vi "Maxi Gauge-RW Sensor Control.vi"(0 "VISA-Ressource in":refnum<visa-resource-name>, 1 "No Control ID´s":string[](array[string])=["no Sensor", "APR/ACR", "TPR"], 2 "Sensor Nr. :":u8(ring) items=["sensor 1", "sensor 2", "sensor 3", "sensor 4", "sensor 5", "sensor 6"], 3 "Control Source ON:":u8(ring) items=["sensor 1", "sensor 2", "sensor 3", "sensor 4", "sensor 5", "sensor 6", "Extern", "Manual", "Hotstart"], 4 "Control Source OFF:":u8(ring) items=["sensor 1", "sensor 2", "sensor 3", "sensor 4", "sensor 5", "sensor 6", "Extern", "Manual", "Hotstart"], 5 "Fehler (Eingang, kein Fehler)":errorcluster, 6 "Node address":i8=-1 min=-1 max=31 step=1, 7 "ON Threshold Set:":dbl=1e-13 min=1e-13 max=41000.0 format="%.2e", 8 "W/R":bool, 9 "OFF Threshold Set:":dbl=1e-13 min=1e-13 max=41000.0 format="%.2e") -> (14 "VISA-Ressource out":refnum<visa-resource-name>, 15 "Control Sensor ON Get:":u8(ring) items=["sensor 1", "sensor 2", "sensor 3", "sensor 4", "sensor 5", "sensor 6", "Extern", "Manual", "Hotstart"], 16 "Control Sensor OFF Get:":u8(ring) items=["sensor 1", "sensor 2", "sensor 3", "sensor 4", "sensor 5", "sensor 6", "Extern", "Manual", "Hotstart"], 17 "ON Threshold Get:":dbl=1e-13 min=1e-13 max=41000.0 format="%.2e", 18 "OFF Threshold Get:":dbl=1e-13 min=1e-13 max=41000.0 format="%.2e", 19 "Fehler (Ausgang)":errorcluster)   [LabVIEW 2012, in "Maxi Gauge.lvlib"]
uses:
  Maxi Gauge.lvlib
panel:
  # "mbar"
  # "mbar"
  # "mbar"
  # "mbar"
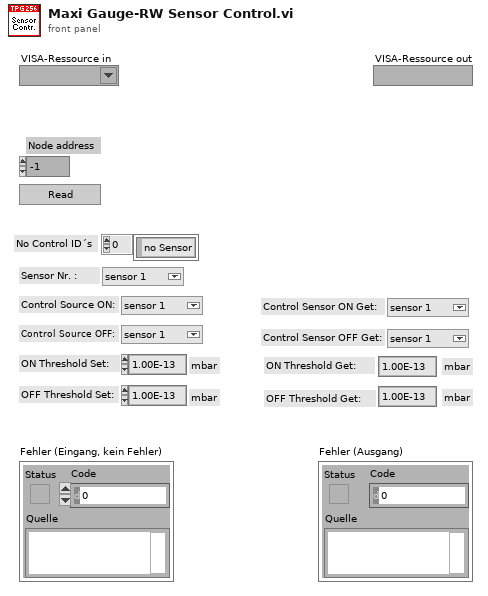
[diagram p1: front panel]
types:
  T1 = cluster{"Sensor 1":string, "Sensor 2":string, "Sensor 3":string, "Sensor 4":string, "Sensor 5":string, "Sensor 6":string}
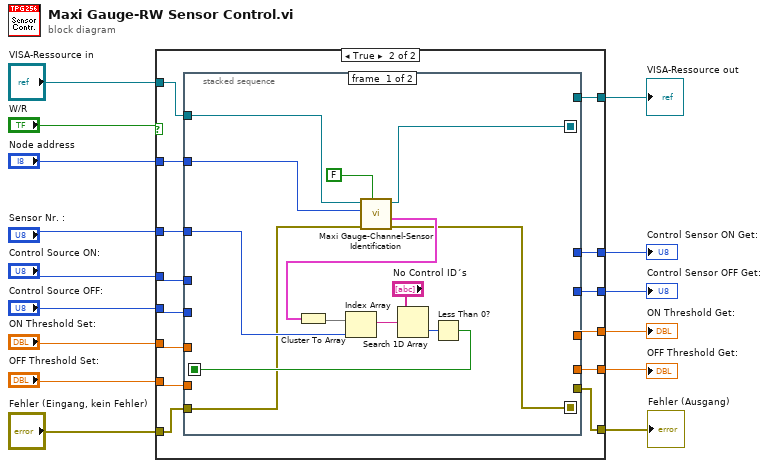
[diagram p0: block diagram]
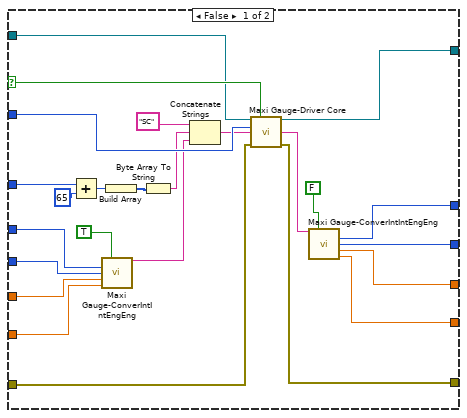
[diagram p2: hidden frame]
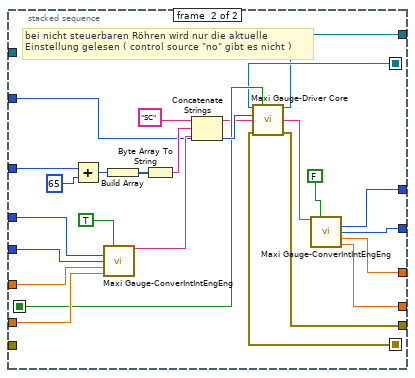
[diagram p3: hidden frame]
diagram:
  n1 = case shown="True" "W/R" {
    selector: "W/R" -> [w21 _]
    tunnel: "Node address" -> [w40 w54]
    tunnel: "Sensor Nr. :" -> [w37 w53]
    tunnel: [w34 w46] -> w7
    tunnel: [w33 w45] -> w8
    tunnel: [w32 w47] -> w9
    tunnel: [w31 w48] -> w10
    tunnel: "OFF Threshold Set:" -> [w27 w49]
    tunnel: "ON Threshold Set:" -> [w26 w50]
    tunnel: "Control Source OFF:" -> [w25 w51]
    tunnel: "Control Source ON:" -> [w24 w52]
    tunnel: "VISA-Ressource in" -> [w19 w44]
    tunnel: [w18 w43] -> w3
    tunnel: "Fehler (Eingang, kein Fehler)" -> [w17 w42]
    tunnel: [w16 w41] -> w1
    frame False {
      n2 = Add(x=w37, y=65) -> (x+y=w38:i32)
      n3 = call "Maxi Gauge-ConverIntIntEngEng.vi"("W/R [W: Int in; Str out ]"=TRUE, "Integer1 in"=w24, "Integer2 in"=w25, "Eng1 in"=w26, "Eng2 in"=w27) -> ("String out"=w28:string)  [unwired: 6 in, 4 out]
      n4 = Build Array(w38) -> (w36:i32[])
      n5 = Byte Array To String(unsigned byte array=w36) -> (string=w35:string)
      n6 = Concatenate Strings("SC" ("Command"), w35, w28) -> (w20:string)
      n7 = call "Maxi Gauge-Driver Core.vi"("VISA-Ressource in"=w19, "Write/Read"=w21, "Node address"=w40, "Command"=w20, "Fehler (Eingang)"=w17) -> ("VISA-Ressource out"=w18:refnum<visa-resource-name>, "String Out"=w30:string, "Fehler (Ausgang)"=w16:errorcluster)  [unwired: 8 in]
      n8 = call "Maxi Gauge-ConverIntIntEngEng.vi"("String in"=w30, "W/R [W: Int in; Str out ]"=FALSE) -> ("Integer1 out"=w31:u8, "Integer2 out"=w32:u8, "Eng1 out"=w33:dbl, "Eng2 out"=w34:dbl)  [unwired: 9 in, 1 out]
    }
    frame True {
      n9 = stacked-sequence {
        seq-local: [w61 _] -> [_ w73]
        seq-local: [w57 _] -> [_ w71]
        seq-local: [w55 _] -> [_ w68]
        tunnel: w54 -> [w59 w83]
        tunnel: w53 -> [w63 w82]
        tunnel: w52 -> [_ w81]
        tunnel: w51 -> [_ w80]
        tunnel: w50 -> [_ w79]
        tunnel: w49 -> [_ w78]
        tunnel: [_ w77] -> w48
        tunnel: [_ w76] -> w47
        tunnel: [_ w75] -> w45
        tunnel: [_ w74] -> w46
        tunnel: w44 -> [w58 _]
        tunnel: [_ w70] -> w43
        tunnel: w42 -> [w56 _]
        tunnel: [_ w69] -> w41
        frame #0 {
          n10 = call "Maxi Gauge-Channel-Sensor Identification.vi"("W/R"=FALSE, "Fehler (Eingang, kein Fehler)"=w56, "Node address"=w59, "VISA-Ressource in"=w58) -> ("Fehler (Ausgang)"=w55:errorcluster, "Get Sensor Identification"=w60:T1, "VISA-Ressource out"=w57:refnum<visa-resource-name>)  [unwired: 4 in, 1 out]
          n11 = Cluster To Array(cluster=w60) -> (array=w64:string[])
          n12 = Index Array(array=w64, index=w63) -> (element=w62:string)
          n13 = Search 1D Array(1D array="No Control ID´s", element=w62) -> (index of element=w65:i32)  [unwired: 1 in]
          n14 = Less Than 0?(x=w65) -> (x < 0?=w61:bool)
        }
        frame #1 {
          # "bei nicht steuerbaren Röhren wird nur die aktuelle\nEinstellung gelesen ( control source \"no\" gibt es nicht )"
          n15 = Add(x=w82, y=65) -> (x+y=w91:i32)
          n16 = call "Maxi Gauge-ConverIntIntEngEng.vi"("W/R [W: Int in; Str out ]"=TRUE, "Integer1 in"=w81, "Integer2 in"=w80, "Eng1 in"=w79, "Eng2 in"=w78) -> ("String out"=w86:string)  [unwired: 6 in, 4 out]
          n17 = Build Array(w91) -> (w90:i32[])
          n18 = Byte Array To String(unsigned byte array=w90) -> (string=w89:string)
          n19 = Concatenate Strings("SC" ("Command"), w89, w86) -> (w72:string)
          n20 = call "Maxi Gauge-Driver Core.vi"("VISA-Ressource in"=w71, "Write/Read"=w73, "Node address"=w83, "Command"=w72, "Fehler (Eingang)"=w68) -> ("VISA-Ressource out"=w70:refnum<visa-resource-name>, "String Out"=w88:string, "Fehler (Ausgang)"=w69:errorcluster)  [unwired: 8 in]
          n21 = call "Maxi Gauge-ConverIntIntEngEng.vi"("String in"=w88, "W/R [W: Int in; Str out ]"=FALSE) -> ("Integer1 out"=w77:u8, "Integer2 out"=w76:u8, "Eng1 out"=w75:dbl, "Eng2 out"=w74:dbl)  [unwired: 9 in, 1 out]
        }
      }
    }
  }
  "Control Sensor ON Get:" <- w10
  "OFF Threshold Get:" <- w7
  "ON Threshold Get:" <- w8
  "Control Sensor OFF Get:" <- w9
  "VISA-Ressource out" <- w3
  "Fehler (Ausgang)" <- w1
